vi "Item.vi"(8 "error in (no error)":errorcluster, 10 "Key":string, 11 "Array In":refnum<class "Array.lvclass">) -> (0 "error out":errorcluster, 1 "Value":refnum<class>, 3 "Array Out":refnum<class "Array.lvclass">)   [LabVIEW 2013, in "LapDog.Collections.v_.Maps.Implementations.lvlib" / "Array.lvclass"]
doc: "Returns a copy of the value associated with the given key.\n\nIf the key does not exist, error 510203 is returned."
uses:
  Array.lvclass
  Array.lvclass/Array.ctl
  LapDog.Collections.Common/LapDog.Collections.v_.Common.lvlib
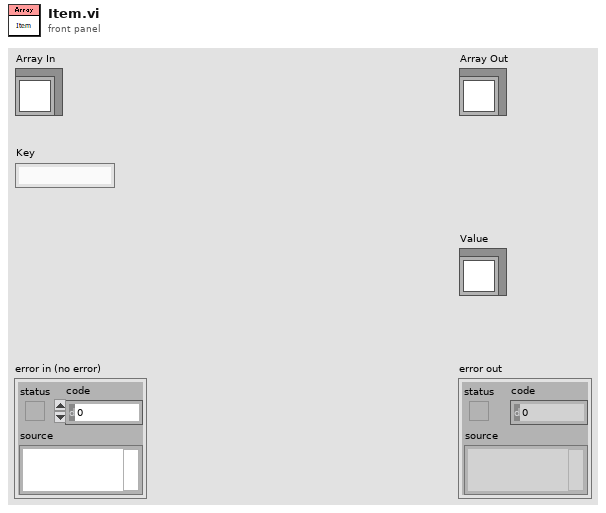
[diagram p1: front panel]
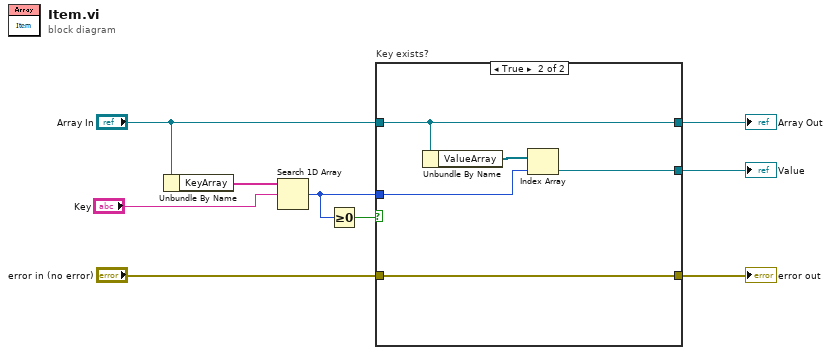
[diagram p0: block diagram]
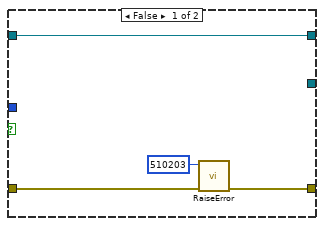
[diagram p2: hidden frame]
diagram:
  n1 = Unbundle By Name("Array In") -> ("KeyArray"=w8:string[])
  n2 = Search 1D Array(1D array=w8, element="Key") -> (index of element=w2:i32)  [unwired: 1 in]
  n3 = Greater Or Equal To 0?(x=w2) -> (x >= 0?=w6:bool)
  n4 = case "Key exists?" shown="True" w6 {
    tunnel: [w12 w17] -> _
    tunnel: "Array In" -> [w12 w17]
    tunnel: "error in (no error)" -> [w11 w13]
    tunnel: [w10 w13] -> w3
    tunnel: w2 -> [_ w15]
    tunnel: [_ w14] -> w1
    frame False {
      n5 = call "RaiseError.vi"("error in (no error)"=w11, "Error Code"=510203) -> ("error out"=w10:errorcluster)  [unwired: 9 in]
    }
    frame True {
      n6 = Unbundle By Name(w17) -> ("ValueArray"=w16:refnum<class>[])
      n7 = Index Array(array=w16, index=w15) -> (element=w14:refnum<class>)
    }
  }
  "error out" <- w3
  "Value" <- w1
  "Array Out" <- "Array In"
